vi "DPT Panel Get Load Info.vi"(2 "file path (dialog if empty)":path, 11 "Error In":errorcluster) -> (6 "Load Type Out":string(combo), 8 "Nominal Load  Weight Out":string(combo), 15 "Error Out":errorcluster)   [LabVIEW 2016, in "File Setup.lvlib"]
uses:
  File Setup.lvlib
  Custom Pallet Controls/Custom Pallet Forward.ctl
  <vilib>/Utility/miscctls.llb/LVComboBoxStrsAndValuesArrayTypeDef.ctl
  <vilib>/Utility/file.llb/Read From Spreadsheet File (string).vi
panel:
  in  "Nominal Load  Weight (Select or Enter Value)":string(combo)
  in  "Load Type (Select or Enter Value)":string(combo)
  in  "Complete":T1
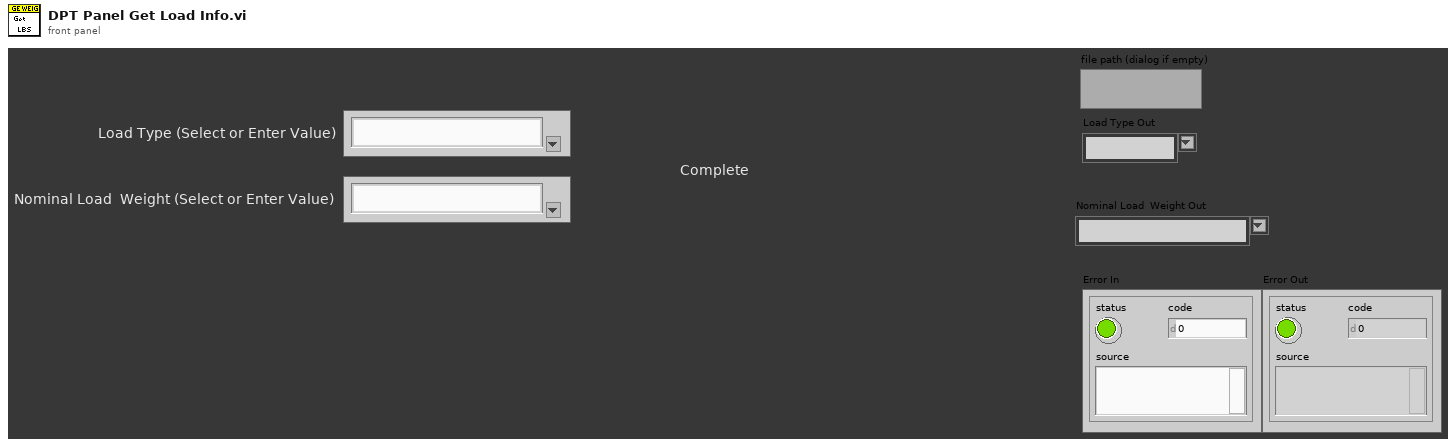
[diagram p1: front panel]
types:
  T1 = typedef "Custom Pallet Forward.ctl" = bool
  T2 = typedef "LVComboBoxStrsAndValuesArrayTypeDef.ctl" = cluster{"String":string, "Value":string}[]
  T3 = enum32{"Invalid", "Standard", "Closed", "Hidden", "Minimized", "Maximized"}
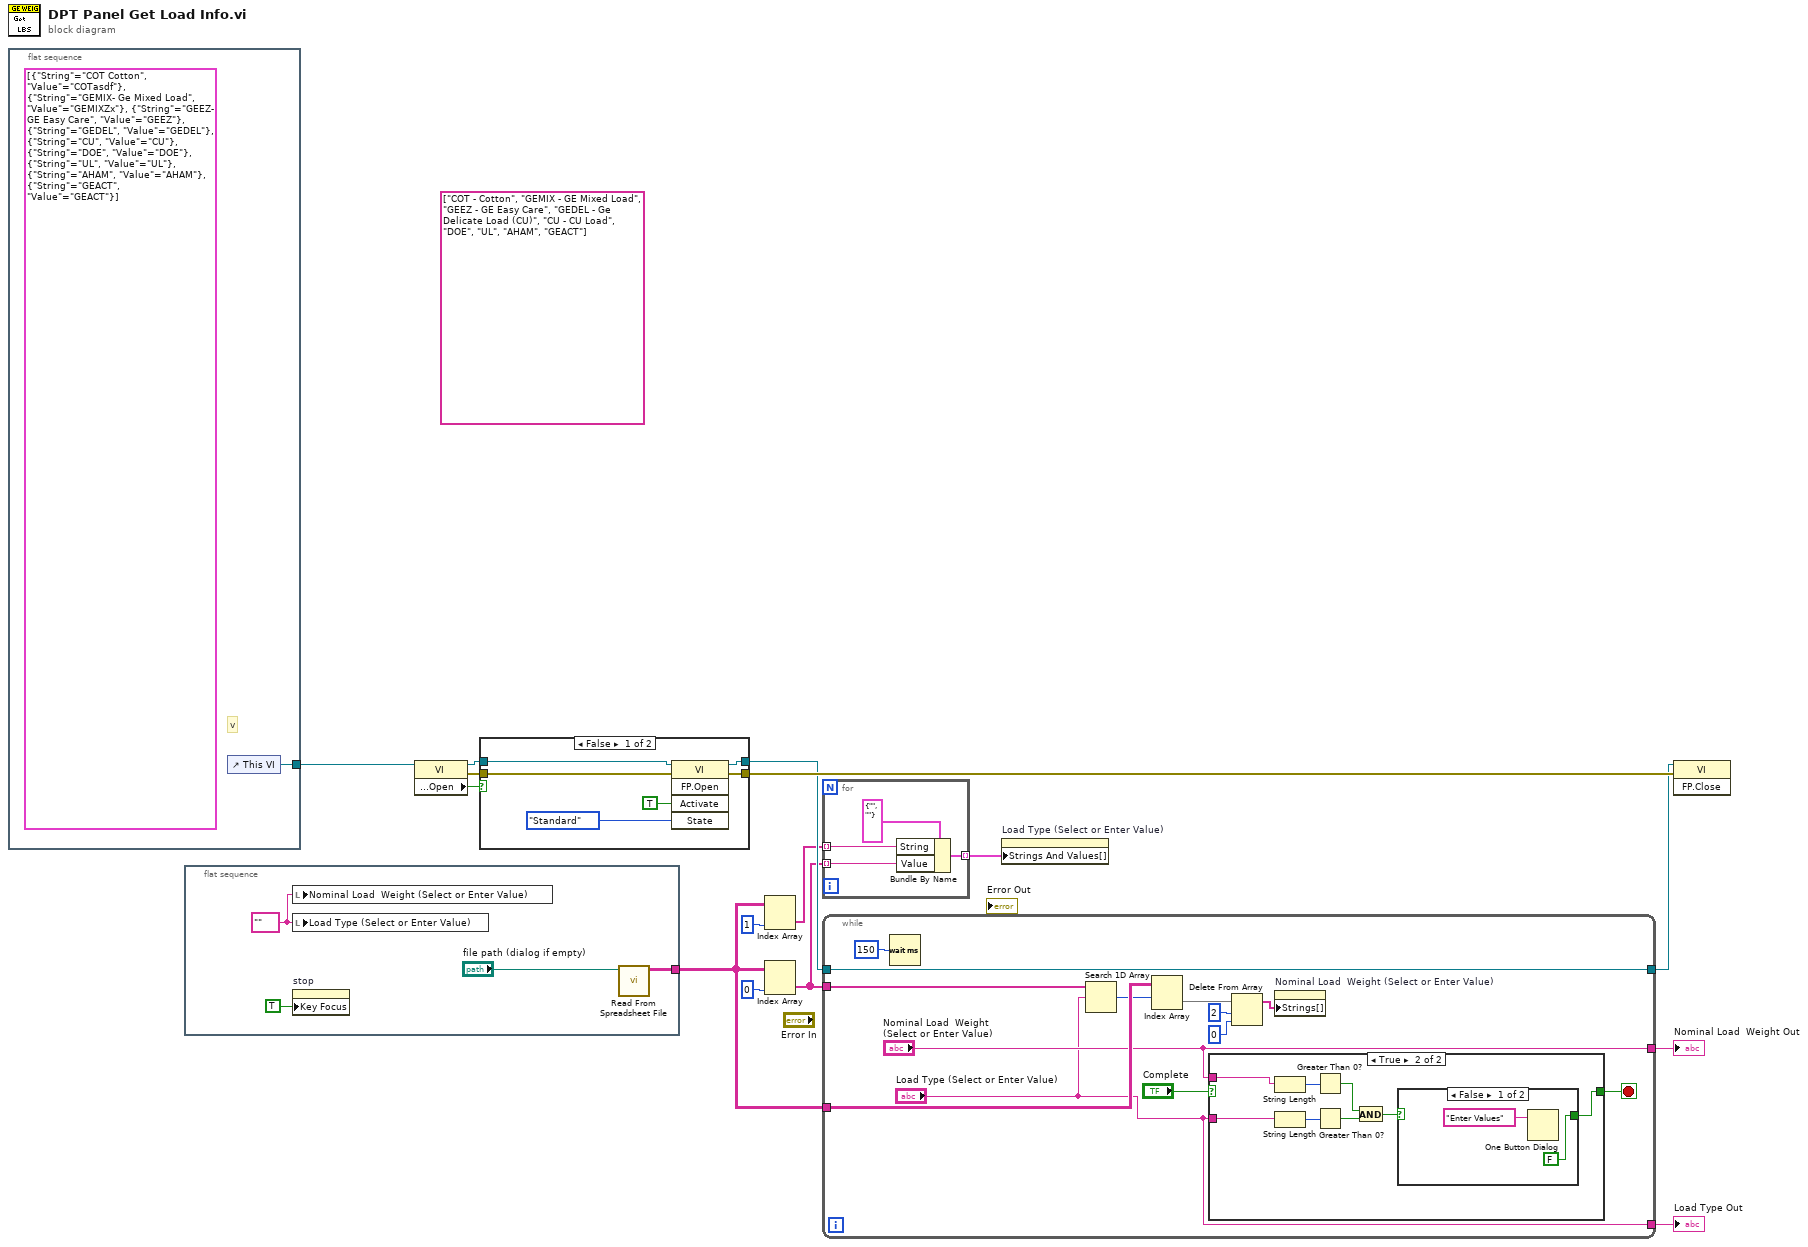
[diagram p0: block diagram]
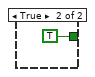
[diagram p4: hidden frame]
diagram:
  (unwired) string[] ["COT - Cotton", "GEMIX - GE Mixed Load", "GEEZ - GE Easy Care", "GEDEL - Ge Delicate Load (CU)", "CU - CU Load", "DOE", "UL", "AHAM", "GEACT"]
  n1 = flat-sequence {
    tunnel: [w16] -> w6
    frame #0 {
      (unwired) T2 [{"String"="COT Cotton", "Value"="COTasdf"}, {"String"="GEMIX- Ge Mixed Load", "Value"="GEMIXZx"}, {"String"="GEEZ- GE Easy Care", "Value"="GEEZ"}, {"String"="GEDEL", "Value"="GEDEL"}, {"String"="CU", "Value"="CU"}, {"String"="DOE", "Value"="DOE"}, {"String"="UL", "Value"="UL"}, {"String"="AHAM", "Value"="AHAM"}, {"String"="GEACT", "Value"="GEACT"}] ("Strings And Values []")
      # "v"
      n2 = control-ref of="This VI"() -> (w16:refnum<vi>)
    }
  }
  n3 = flat-sequence {
    tunnel: [w18] -> w3
    frame #0 {
      w20 = "" ("Load Type (Select or Enter Value)")
      n4 = local write "Nominal Load  Weight (Select or Enter Value)"(w20) -> ()
      n5 = local write "Load Type (Select or Enter Value)"(w20) -> ()
      n6 = property on="stop" class="Bool"("Key Focus"=TRUE) -> ()  [unwired: 2 in, 2 out]
      n7 = call-poly <vilib>:"Read From Spreadsheet File.vi"("file path (dialog if empty)"="file path (dialog if empty)") -> ("all rows"=w18:string[][])  [unwired: 6 in, 4 out]
    }
  }
  n8 = property class="VI"(reference=w6) -> (reference out=w8:refnum<vi>, error out=w9:errorcluster, "Front Panel.Open"=w7:bool)  [unwired: 1 in]
  n9 = case shown="False" w7 {
    tunnel: [w24 w28] -> w12
    tunnel: w9 -> [w23 w28]
    tunnel: w8 -> [w22 w27]
    tunnel: [w21 w27] -> w10
    frame False {
      n10 = invoke class="VI" method="FP.Open"(reference=w22, error in=w23, "Activate"=TRUE, "State"=T3."Standard") -> (reference out=w21:refnum<vi>, error out=w24:errorcluster)  [unwired: 1 in, 3 out]
    }
    frame True {
    }
  }
  n11 = Index Array(array=w3, index (col)=1 ("disabled index (col)")) -> (element=w2:string[])  [unwired: 1 in]
  n12 = Index Array(array=w3, index (col)=0 ("disabled index (col)")) -> (element=w5:string[])  [unwired: 1 in]
  n13 = for {
    tunnel: w5 -> [w32] mode=indexing
    tunnel: w2 -> [w31] mode=indexing
    tunnel: [w29] -> w1 mode=indexing
    n14 = Bundle By Name(cluster=cluster{"String":string, "Value":string} {"String"="", "Value"=""} ("Cluster"), "String"=w31, "Value"=w32) -> (w29:cluster{"String":string, "Value":string})
  }
  n15 = while {
    tunnel: w5 -> [w44]
    tunnel: ["Load Type (Select or Enter Value)"] -> w14
    tunnel: w3 -> [w43]
    tunnel: ["Nominal Load  Weight (Select or Enter Value)"] -> w13
    tunnel: [w37] -> w11
    tunnel: w10 -> [w37]
    stop <- w33 stop-if-true
    n16 = Wait (ms)(milliseconds to wait=u32 150) -> ()  [unwired: 1 out]
    n17 = Search 1D Array(1D array=w44, element="Load Type (Select or Enter Value)") -> (index of element=w42:i32)  [unwired: 1 in]
    n18 = Index Array(array=w43, index (row)=w42) -> (element=w41:string[])  [unwired: 1 in]
    n19 = case shown="True" "Complete" {
      selector: "Complete" -> [w46 _]
      tunnel: "Nominal Load  Weight (Select or Enter Value)" -> [_ w50]
      tunnel: "Load Type (Select or Enter Value)" -> [_ w49]
      tunnel: [w46 w47] -> w33
      frame False {
      }
      frame True {
        n20 = String Length(string=w50) -> (length=w54:i32)
        n21 = String Length(string=w49) -> (length=w53:i32)
        n22 = Greater Than 0?(x=w54) -> (x > 0?=w52:bool)
        n23 = Greater Than 0?(x=w53) -> (x > 0?=w51:bool)
        n24 = And(x=w52, y=w51) -> (x .and. y?=w48:bool)
        n25 = case shown="False" w48 {
          tunnel: [FALSE TRUE] -> w47
          frame False {
            n26 = One Button Dialog(message="Enter Values") -> ()  [unwired: 1 in, 1 out]
          }
          frame True {
          }
        }
      }
    }
    n27 = Delete From Array(array=w41, length=2, index=0) -> (array with subset deleted=w38:string[])  [unwired: 1 out]
    n28 = property on="Nominal Load  Weight (Select or Enter Value)" class="CmbBox"("Strings[]"=w38) -> ()  [unwired: 2 in, 2 out]
  }
  "Load Type Out" <- w14
  "Nominal Load  Weight Out" <- w13
  n29 = property on="Load Type (Select or Enter Value)" class="CmbBox"("Strings And Values[]"=w1) -> ()  [unwired: 2 in, 2 out]
  n30 = invoke class="VI" method="FP.Close"(reference=w11, error in=w12) -> ()  [unwired: 1 in, 3 out]
